vi "Show Ephys.vi"(11 "Array":dbl[][](array[numeric])) -> ()   [LabVIEW 2018]
panel:
  out "Waveform Graph 6":dbl[](graph)
  out "Waveform Graph 5":dbl[](graph)
  out "Waveform Graph 4":dbl[](graph)
  out "Waveform Graph 3":dbl[](graph)
  out "Waveform Graph 2":dbl[](graph)
  out "Waveform Graph 1":dbl[](graph)
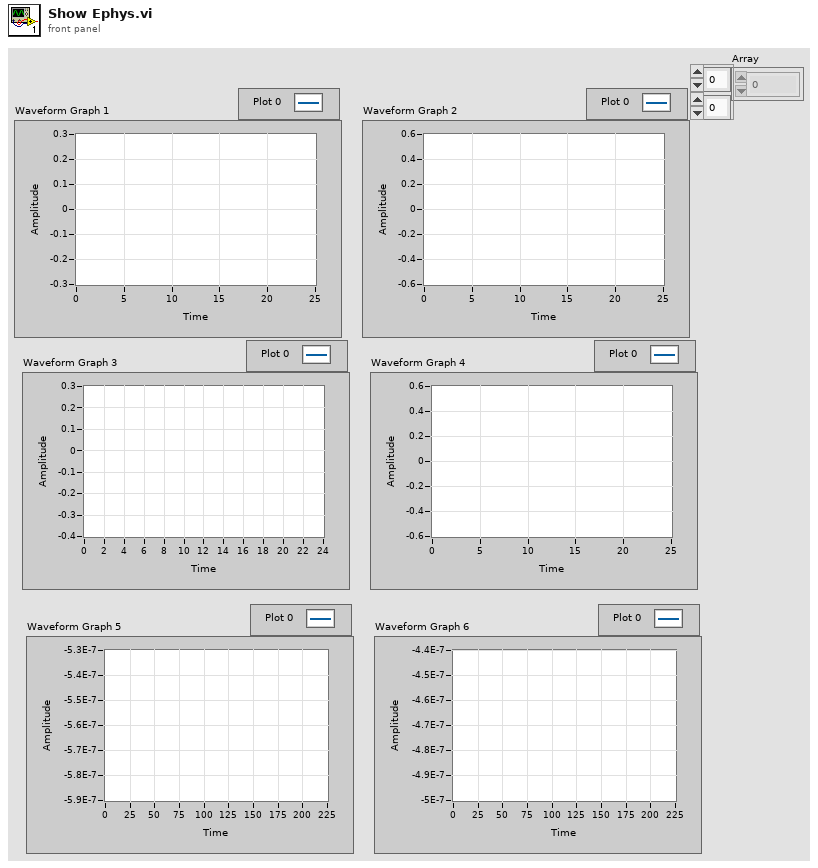
[diagram p1: front panel]
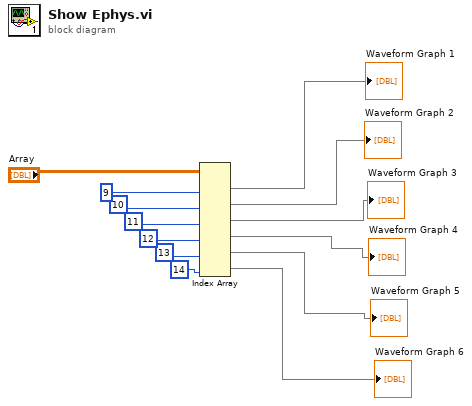
[diagram p0: block diagram]
diagram:
  n1 = Index Array(array="Array", index (col) #1=9 ("disabled index (col)"), index (col) #2=10 ("disabled index (col)"), index (col) #3=11 ("disabled index (col)"), index (col) #4=12 ("disabled index (col)"), index (col) #5=13 ("disabled index (col)"), index (col) #6=14 ("disabled index (col)")) -> (element #1=→"Waveform Graph 1":dbl[], element #2=→"Waveform Graph 2":dbl[], element #3=→"Waveform Graph 3":dbl[], element #4=→"Waveform Graph 4":dbl[], element #5=→"Waveform Graph 5":dbl[], element #6=→"Waveform Graph 6":dbl[])  [unwired: 6 in]
